vi "mysql写入.vi"() -> ()   [LabVIEW 2020]
uses:
  <vilib>/addons/database/Connection.llb/DB Tools Open Connec (Path).vi
  <vilib>/addons/database/Connection.llb/Conn Execute.vi
  <vilib>/addons/database/NI_Database_API.lvlib
panel:
  out "error out":errorcluster
  in  "connection information":path
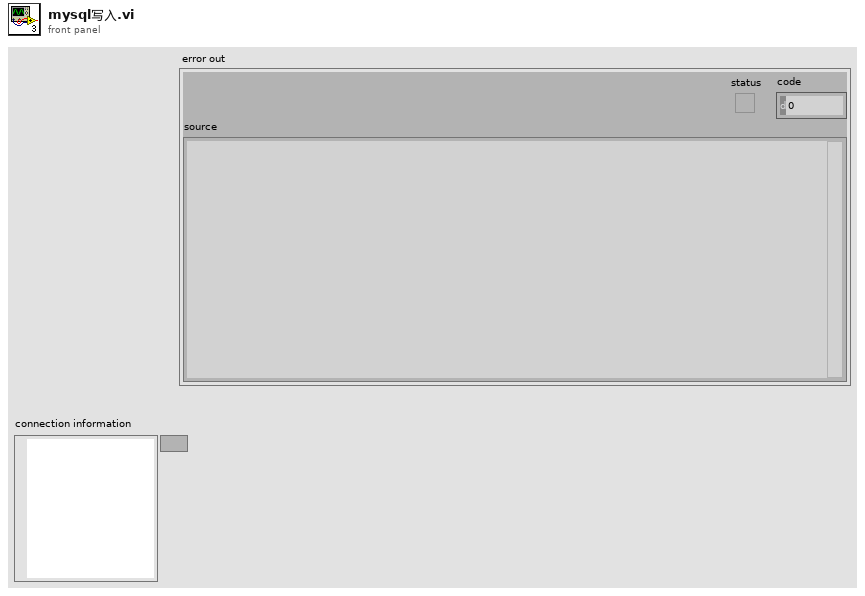
[diagram p1: front panel]
types:
  T1 = typedef "NI_Database_API.lvlib/Conn ObjectReference.ctl" = refnum<k1>
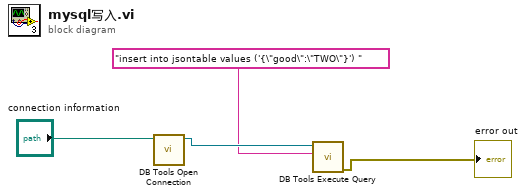
[diagram p0: block diagram]
diagram:
  n1 = call-poly <vilib>:"DB Tools Open Connection.vi"("connection information"="connection information") -> ("connection reference"=w3:T1)  [unwired: 7 in, 1 out]
  n2 = call-poly <vilib>:"DB Tools Execute Query.vi"("SQL query"="insert into jsontable values ('{\"good\":\"TWO\"}') ", "connection reference"=w3) -> ("error out"=→"error out":errorcluster)  [unwired: 6 in, 1 out]
